vi "Fault View.vi"(10 "User Events in":refnum<class "User Events.lvclass">) -> ()   [LabVIEW 2016, in "FAMT Views.lvlib"]
uses:
  FAMT Views.lvlib
  User Events/User Events.lvclass
  User Events/User Events.lvclass/User Events.ctl
  Typedefs/StateTypes.ctl
  <vilib>/Utility/error.llb/DialogType.ctl
  Typedefs/FAMT Typedefs.lvlib
panel:
  out "Fault":string
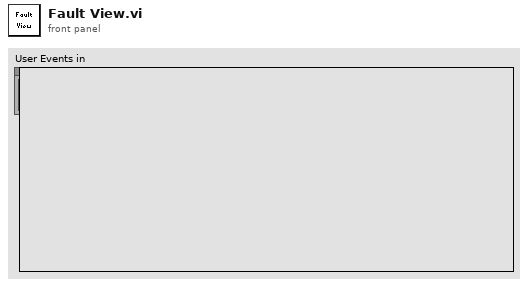
[diagram p1: front panel]
types:
  T1 = typedef "FAMT Typedefs.lvlib/Publish Data Events.ctl" = cluster{"State":refnum<user-event>, "ErrorCode":refnum<user-event>, "Scan Progress":refnum<user-event>, "All Test Status":refnum<user-event>}
  T2 = cluster{"Event Registration Refnum":refnum<event-registration>, "Event Registration Refnum":refnum<event-registration>}
  T3 = typedef "FAMT Typedefs.lvlib/StateTypes.ctl" = enum16{"Offline State", "Fault State", "Standby State", "Disabled State", "Enabled State", "Wait For User Input State", "Test Actuator State"}
  T4 = typedef "DialogType.ctl" = u16
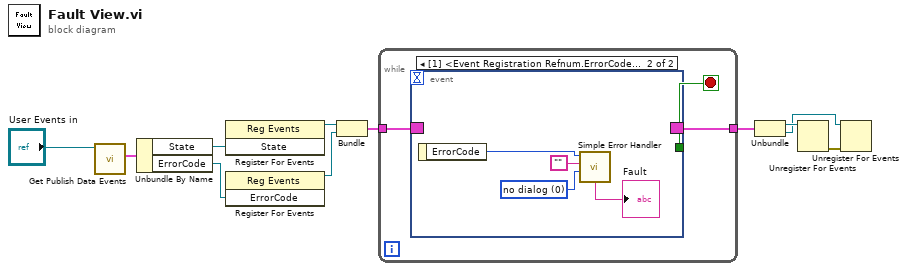
[diagram p0: block diagram]
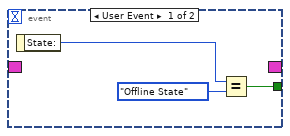
[diagram p2: hidden frame]
diagram:
  n1 = call "Get Publish Data Events.vi"("UserEvents in"="User Events in") -> ("Publish Data Events"=w9:T1)  [unwired: 9 in, 1 out]
  n2 = Unbundle By Name(w9) -> ("State"=w10:refnum<user-event>, "ErrorCode"=w4:refnum<user-event>)
  n3 = register-events(w10) -> (reference out=w11:refnum<event-registration>)  [unwired: 2 in, 1 out]
  n4 = register-events(w4) -> (reference out=w3:refnum<event-registration>)  [unwired: 2 in, 1 out]
  n5 = Bundle("Event Registration Refnum"=w11, "Event Registration Refnum"=w3) -> (w8:T2)  [unwired: 1 in]
  n6 = while {
    tunnel: w8 -> [w14]
    tunnel: [w13] -> w7
    stop <- w12 stop-if-true
    n7 = event shown="[1] <Event Registration Refnum.ErrorCode>: User Event" {
      selector: w14 -> [_ _]
      dyn-events: [_ _] -> w13
      timeout: _ -> [_ _]
      tunnel: [w16 _] -> w12
      event User Event {
        n8 = event-data() -> ("State:"=w15:T3)  [unwired: 1 in]
        n9 = Equal?(x=w15, y=StateTypes."Offline State") -> (x = y?=w16:bool)
      }
      event User Event {
        w21 = T4 0 items=["no dialog", "OK message", "continue or stop message", "OK message + warnings", "continue/stop + warnings"] ("type of dialog (OK msg:1)")
        n10 = event-data() -> ("ErrorCode"=w19:i32)  [unwired: 1 in]
        n11 = call <vilib>:"Simple Error Handler.vi"("error code (no error:0)"=w19, "error source (\" \")"="", "type of dialog (OK msg:1)"=w21) -> ("message"=→"Fault":string)  [unwired: 2 in, 4 out]
      }
    }
  }
  n12 = Unbundle(w7) -> ("Event Registration Refnum"=w6:refnum<event-registration>, "Event Registration Refnum"=w2:refnum<event-registration>)
  n13 = Unregister For Events(event registration refnum=w6) -> (error out=w1:errorcluster)  [unwired: 1 in]
  n14 = Unregister For Events(event registration refnum=w2, error in=w1) -> ()  [unwired: 1 out]
